vi "edit_entry.vi"(4 "Converted":dbl[](array[numeric]), 5 "Raw":dbl[](array[numeric]), 6 "Offset":dbl, 7 "error in":errorcluster, 8 "Average":dbl, 9 "Label":string, 10 "Active Analog Data In":T1[](array[typedef])) -> (0 "error out":errorcluster, 3 "Active Analog Data Out":T1[](array[typedef]))   [LabVIEW 2017]
uses:
  analog_data.ctl
panel:
  in  "Analog Data":T1
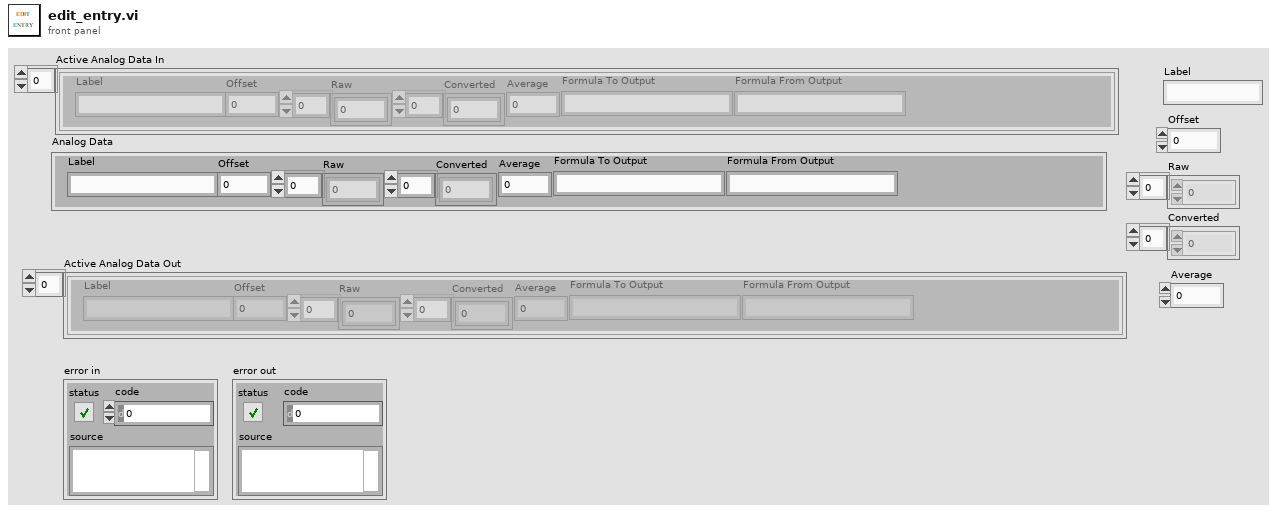
[diagram p1: front panel]
types:
  T1 = typedef "analog_data.ctl" = cluster{"Label":string, "Offset":dbl, "Raw":dbl[], "Converted":dbl[], "Average":dbl, "Formula To Output":string, "Formula From Output":string}
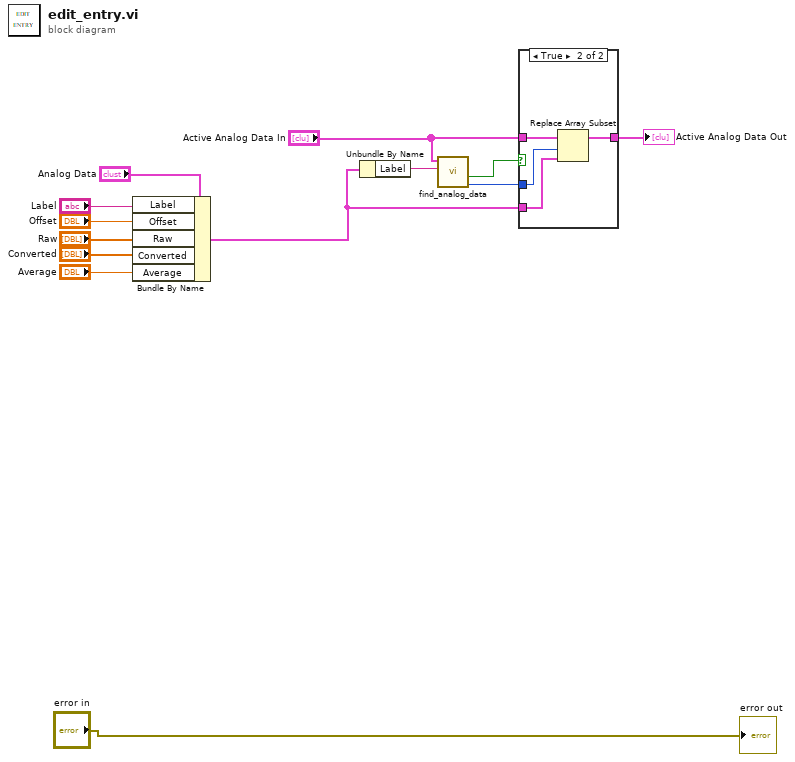
[diagram p0: block diagram]
diagram:
  n1 = Bundle By Name(cluster="Analog Data", "Label"="Label", "Offset"="Offset", "Raw"="Raw", "Converted"="Converted", "Average"="Average") -> (w6:T1)
  n2 = Unbundle By Name(w6) -> ("Label"=w10:string)
  n3 = call "find_analog_data.vi"("Needle"=w10, "Haystack"="Active Analog Data In") -> ("Index"=w8:i32, "Found?"=w9:bool)  [unwired: 7 in, 1 out]
  n4 = case shown="True" w9 {
    tunnel: [w14 w18] -> w13
    tunnel: "Active Analog Data In" -> [w14 w17]
    tunnel: w6 -> [_ w16]
    tunnel: w8 -> [_ w15]
    frame False {
    }
    frame True {
      n5 = Replace Array Subset(array=w17, new element=w16, index=w15) -> (w18:T1[])
    }
  }
  "Active Analog Data Out" <- w13
  "error out" <- "error in"
